vi "Agilent 34970 Read Scanlist.vi"(2 "error in (no error)":errorcluster, 3 "VISA Resource Name":refnum<visa-resource-name>) -> (0 "error out":errorcluster, 1 "Output Data (Numbers Only)":dbl[](array[numeric]))   [LabVIEW 2016]
uses:
  Agilent 34970.lvlib
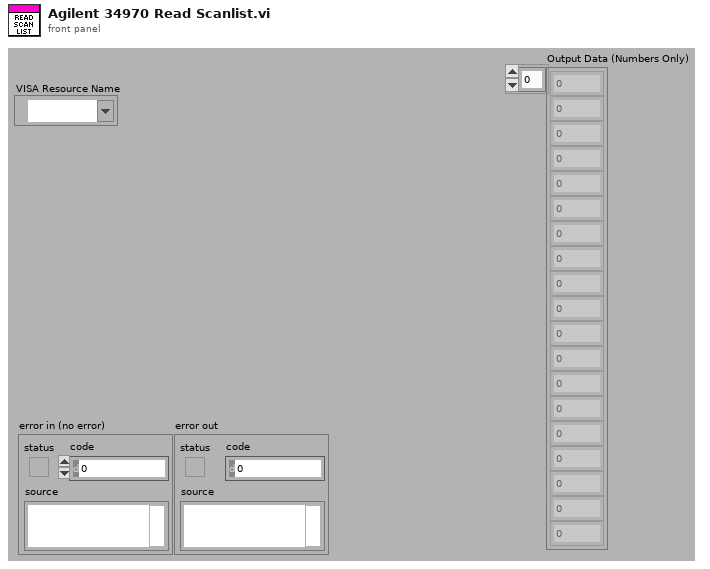
[diagram p1: front panel]
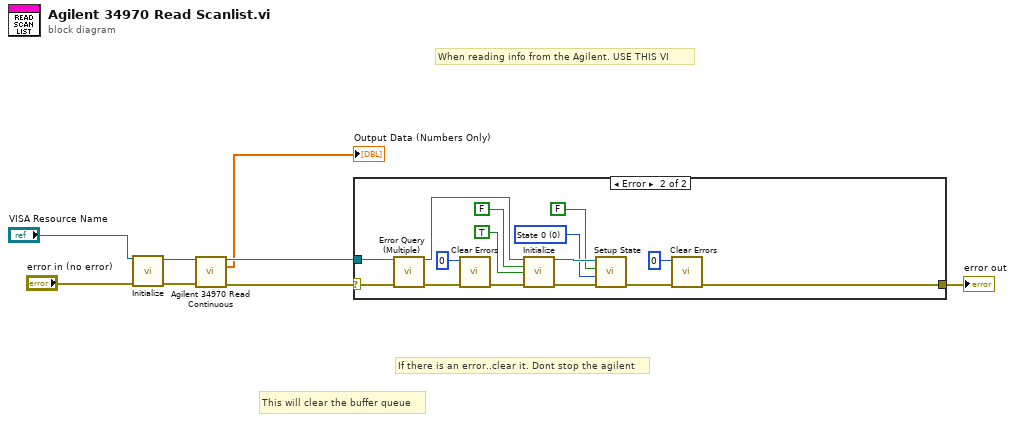
[diagram p0: block diagram]
diagram:
  # "When reading info from the Agilent. USE THIS VI"
  # "If there is an error..clear it. Dont stop the agilent"
  # "This will clear the buffer queue"
  n1 = call "Initialize.vi"("VISA Resource Name"="VISA Resource Name", "error in (no error)"="error in (no error)") -> ("VISA Resource Name Out"=w4:refnum<visa-resource-name>, "error out"=w5:errorcluster)  [unwired: 12 in]
  n2 = call "Agilent 34970 Read Continuous.vi"("VISA Resource Name"=w4, "error in (no error)"=w5) -> ("VISA resource name out"=w3:refnum<visa-resource-name>, "Output Array"=→"Output Data (Numbers Only)":dbl[], "error out"=w2:errorcluster)  [unwired: 10 in, 1 out]
  n3 = case shown="Error" w2 {
    selector: w2 -> [w9 w21]
    tunnel: w3 -> [_ w23]
    tunnel: [w9 w11] -> w6
    frame No Error {
    }
    frame Error {
      w13 = u16 0 items=["State 0", "State 1", "State 2", "State 3", "State 4", "State 5", "Preset State"] ("Setup State (6:Preset)")
      n4 = call "Error Query (Multiple).vi"("VISA Resource Name"=w23, "error in (no error)"=w21) -> ("VISA Resource Name Out"=w15:refnum<visa-resource-name>, "error out"=w22:errorcluster)  [unwired: 10 in, 2 out]
      n5 = call <vilib>:"Clear Errors.vi"("error in (no error)"=w22, "specific error code to clear (0: all)"=0) -> ("error out"=w16:errorcluster)  [unwired: 4 in, 1 out]
      n6 = call "Initialize.vi"("VISA Resource Name"=w15, "ID Query (T: Check)"=FALSE, "Reset (T: Reset)"=TRUE, "error in (no error)"=w16) -> ("VISA Resource Name Out"=w20:refnum<visa-resource-name>, "error out"=w19:errorcluster)  [unwired: 10 in]
      n7 = call "Setup State.vi"("error in (no error)"=w19, "Setup State (6:Preset)"=w13, "Recall/Save (F=Recall)"=FALSE, "VISA Resource Name"=w20) -> ("error out"=w12:errorcluster)  [unwired: 6 in, 1 out]
      n8 = call <vilib>:"Clear Errors.vi"("error in (no error)"=w12, "specific error code to clear (0: all)"=0) -> ("error out"=w11:errorcluster)  [unwired: 4 in, 1 out]
    }
  }
  "error out" <- w6
